vi "GetHostInControl.vi"(8 "error in (no error)":errorcluster, 11 "SM1000-control in":T2) -> (0 "error out":errorcluster, 2 "Host in control":T1=enum."Pendant", 3 "SM1000-control out":T2)   [LabVIEW 2013, in "EC1000-control.lvlib" / "SM1000-control.lvclass"]
doc: "Returns the current host interface that has exclusive control of the EC1000.\n\n\"Pendant\": Control has been granted to the pendant interface.\n\"LANStream\": Control has been granted to the streaming LAN interface.\n\"LAN\": Control has been granted to the LAN remote control interface.\n\nCommand: \"GetHostInControl\" or 5\nReturns: \"Pendant\"/\"LANStream\"/\"LAN\""
uses:
  SM1000-control.lvclass
  Object-reference.ctl
  Hosts.ctl
  SM1000-control.lvclass/SM1000-control.ctl
  Custom-errors.ctl
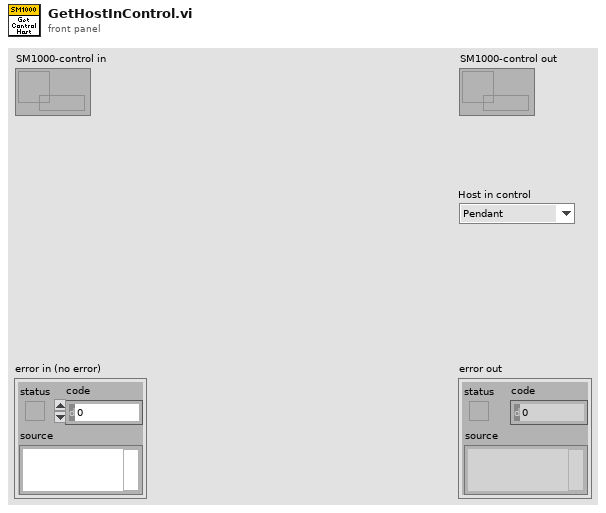
[diagram p1: front panel]
types:
  T1 = typedef "EC1000-control.lvlib/SM1000-control.lvclass/Hosts.ctl" = enum16{"None", "Pendant", "LANStream", "LAN"}
  T2 = typedef "EC1000-control.lvlib/SM1000-control.lvclass/Object-reference.ctl" = refnum<data-value>
  T3 = typedef "EC1000-control.lvlib/SM1000-control.lvclass/Custom-errors.ctl" = enum16{"No error", "Not implemented", "Command not recognized", "Invalid input", "No connection", "Timeout", "Resource not loaded"}
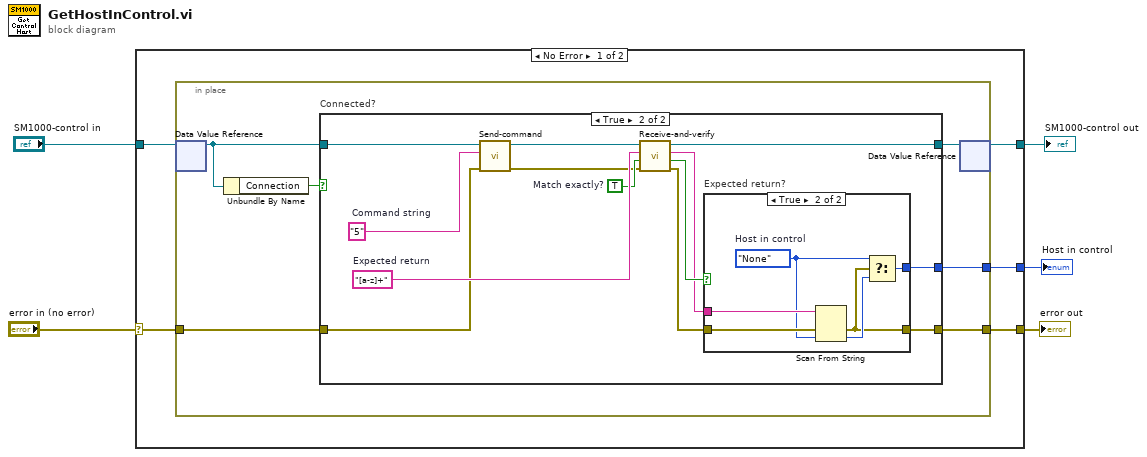
[diagram p0: block diagram]
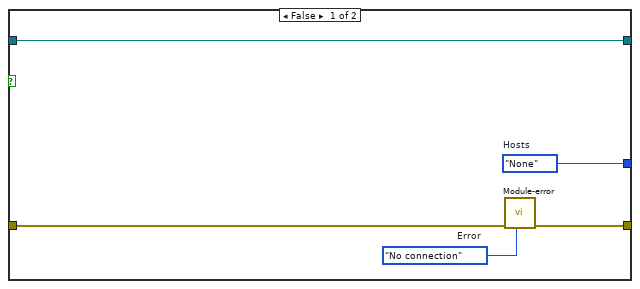
[diagram p2: hidden frame]
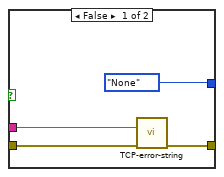
[diagram p3: hidden frame]
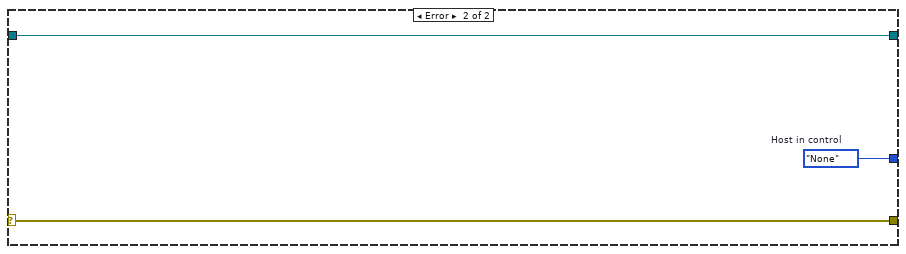
[diagram p4: hidden frame]
diagram:
  n1 = case shown="No Error" "error in (no error)" {
    selector: "error in (no error)" -> [w8 w47]
    tunnel: [w7 w47] -> w4
    tunnel: [w9 w46] -> w2
    tunnel: "SM1000-control in" -> [w10 w46]
    tunnel: [w6 w45] -> w1
    frame No Error {
      n2 = in-place {
        in-place-border: w8 -> [w16]
        in-place-border: [w13] -> w7
        in-place-border: [w11] -> w6
        n3 = in-place-dvr #1(w10) -> (w14:refnum<class "SM1000-control.lvclass">)  [unwired: 1 out]
        n4 = Unbundle By Name(w14) -> ("Connection"=w15:bool)
        n5 = case "Connected?" shown="True" w15 {
          tunnel: w16 -> [w21 w26]
          tunnel: w14 -> [w19 w34]
          tunnel: [w20 w24] -> w13
          tunnel: [w19 w23] -> w12
          tunnel: [w18 w22] -> w11
          frame False {
            w17 = Custom-errors."No connection"  # Error
            w18 = Hosts."None"  # Hosts
            n6 = call "Module-error.vi"("Error"=w17, "error in (no error)"=w21) -> ("error out"=w20:errorcluster)  [unwired: 9 in]
          }
          frame True {
            w30 = TRUE  # Match exactly?
            w31 = "[a-z]+"  # Expected return
            w32 = "5"  # Command string
            n7 = call "Send-command.vi"("error in (no error)"=w26, "Command string"=w32, "SM1000-control in"=w34) -> ("error out"=w29:errorcluster, "SM1000-control out"=w33:refnum<class "SM1000-control.lvclass">)  [unwired: 7 in]
            n8 = call "Receive-and-verify.vi"("error in (no error)"=w29, "Match exactly?"=w30, "Expected return string"=w31, "SM1000-control in"=w33) -> ("error out"=w25:errorcluster, "Verified?"=w28:bool, "Return string"=w27:string, "SM1000-control out"=w23:refnum<class "SM1000-control.lvclass">)  [unwired: 4 in]
            n9 = case "Expected return?" shown="True" w28 {
              tunnel: w27 -> [w38 w43]
              tunnel: w25 -> [w37 w44]
              tunnel: [w36 w40] -> w24
              tunnel: [Hosts."None" ("Host in control") w42] -> w22
              frame False {
                n10 = call "TCP-error-string.vi"("error in (no error)"=w37, "Retun code"=w38) -> ("error out"=w36:errorcluster)  [unwired: 9 in]
              }
              frame True {
                w39 = Hosts."None"  # Host in control
                n11 = Scan From String(input string=w43, error in=w44, default 1=w39) -> (error out=w40:errorcluster, output 1=w41:T1)  [unwired: 2 in, 2 out]
                n12 = Select(t=w39, s=w40, f=w41) -> (s? t:f=w42:T1)
              }
            }
          }
        }
        n13 = in-place-dvr #1(w12) -> (w9:T2)  [unwired: 1 out]
      }
    }
    frame Error {
      w45 = Hosts."None"  # Host in control
    }
  }
  "error out" <- w4
  "SM1000-control out" <- w2
  "Host in control" <- w1
